vi "WPI_CounterWARNDisabledType.vi"() -> (1 "DisabledType":errorcluster)   [LabVIEW 2017]
doc: "This software is licensed. Open the labview\\readme\\WPI Robotics Library Open Source License.txt file for more information."
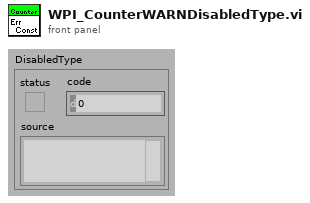
[diagram p1: front panel]
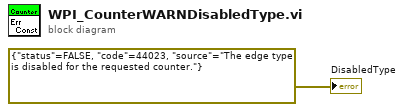
[diagram p0: block diagram]
diagram:
  "DisabledType" <- errorcluster {"status"=FALSE, "code"=44023, "source"="The edge type is disabled for the requested counter."} ("error out 2")
